vi "Write Value at Path(Array).vi"(8 "error in (no error)":errorcluster, 9 "Element in":variant, 10 "Path in":string[](array[string]), 11 "Variant in":variant) -> (0 "error out":errorcluster, 3 "Variant out":variant)   [LabVIEW 2020, in "Variant Data Manipulation.lvlib"]
uses:
  Variant Data Manipulation.lvlib
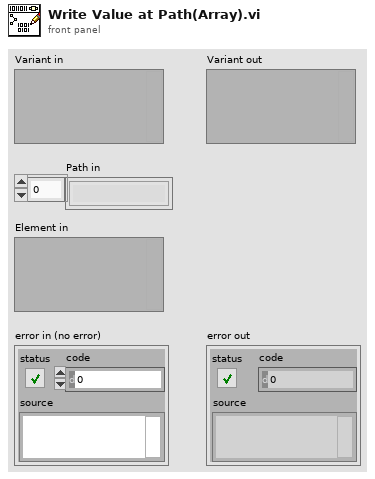
[diagram p1: front panel]
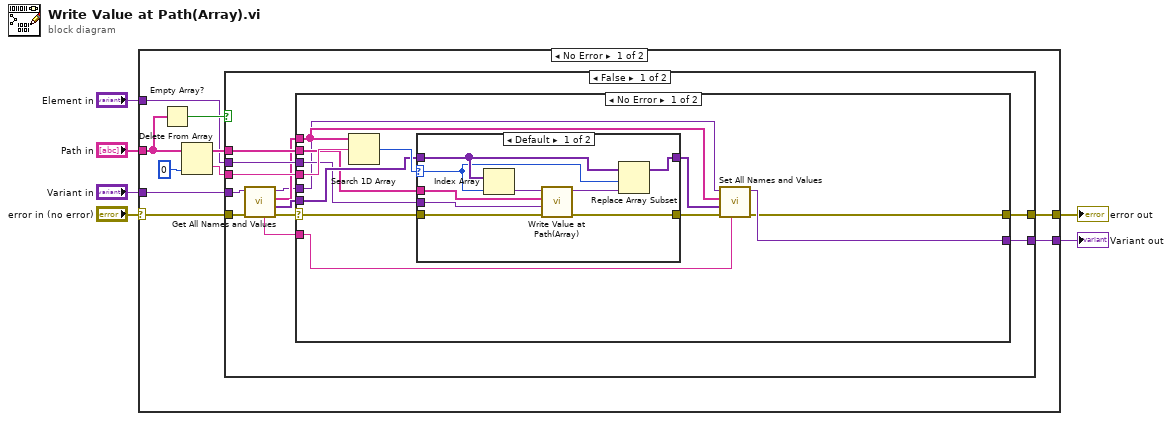
[diagram p0: block diagram]
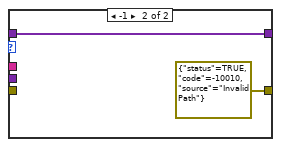
[diagram p2: hidden frame]
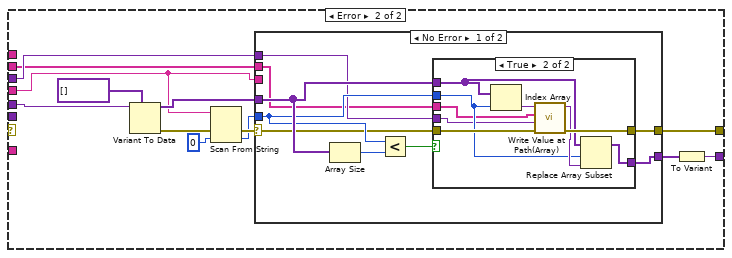
[diagram p3: hidden frame]
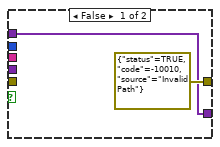
[diagram p4: hidden frame]
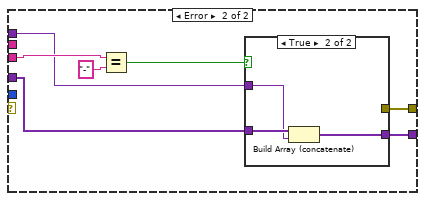
[diagram p5: hidden frame]
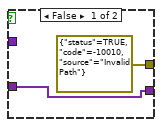
[diagram p6: hidden frame]
diagram:
  n1 = case shown="No Error" "error in (no error)" {
    selector: "error in (no error)" -> [w15 w101]
    tunnel: "Path in" -> [w11 _]
    tunnel: "Variant in" -> [w16 w100]
    tunnel: [w7 w101] -> w4
    tunnel: [w8 w100] -> w2
    tunnel: "Element in" -> [w9 _]
    frame No Error {
      n2 = Empty Array?(array=w11) -> (empty?=w10:bool)
      n3 = Delete From Array(array=w11, index=0) -> (deleted portion=w14:string, array with subset deleted=w12:string[])  [unwired: 1 in]
      n4 = case shown="False" w10 {
        tunnel: w16 -> [w28 _]
        tunnel: w15 -> [w27 w99]
        tunnel: w14 -> [w24 _]
        tunnel: w12 -> [w23 _]
        tunnel: w9 -> [w22 w98]
        tunnel: [w18 w98] -> w8
        tunnel: [w17 w99] -> w7
        frame False {
          n5 = call "Get All Names and Values.vi"("error in"=w27, "Cluster in"=w28) -> ("error out"=w26:errorcluster, "Values"=w25:variant[], "Element Names"=w21:string[], "Cluster out"=w20:variant, "Cluster Name"=w19:string)  [unwired: 5 in]
          n6 = case shown="No Error" w26 {
            selector: w26 -> [w39 _]
            tunnel: w20 -> [w29 w62]
            tunnel: w24 -> [w38 w53]
            tunnel: w21 -> [w34 _]
            tunnel: w25 -> [w40 _]
            tunnel: w23 -> [w37 w57]
            tunnel: w22 -> [w36 w58]
            tunnel: w19 -> [w35 _]
            tunnel: [w31 w56] -> w18
            tunnel: [w30 w54] -> w17
            frame No Error {
              n7 = Search 1D Array(1D array=w34, element=w38) -> (index of element=w41:i32)  [unwired: 1 in]
              n8 = case shown="Default" w41 {
                selector: w41 -> [w46 _]
                tunnel: [w48 errorcluster {"status"=TRUE, "code"=-10010, "source"="Invalid Path"} ("error IO")] -> w32
                tunnel: w40 -> [w47 w51]
                tunnel: w39 -> [w49 _]
                tunnel: w37 -> [w43 _]
                tunnel: w36 -> [w42 _]
                tunnel: [w44 w51] -> w33
                frame Default {
                  n9 = Index Array(array=w47, index=w46) -> (element=w50:variant)
                  n10 = call "Write Value at Path(Array).vi"("error in (no error)"=w49, "Element in"=w42, "Path in"=w43, "Variant in"=w50) -> ("error out"=w48:errorcluster, "Variant out"=w45:variant)  [unwired: 6 in]
                  n11 = Replace Array Subset(array=w47, new element=w45, index=w46) -> (w44:variant[])
                }
                frame -1 {
                }
              }
              n12 = call "Set All Names and Values.vi"("Cluster Name"=w35, "error in"=w32, "values"=w33, "Element Names"=w34, "Cluster in"=w29) -> ("error out"=w30:errorcluster, "Cluster out"=w31:variant)  [unwired: 5 in]
            }
            frame Error {
              n13 = Variant To Data(type=variant[] [], Variant=w62) -> (data=w60:variant[], error out=w59:errorcluster)  [unwired: 1 in]
              n14 = Scan From String(input string=w53, error in=w59, default 1=0 ("default value 1")) -> (error out=w64:errorcluster, output 1=w63:i32)  [unwired: 2 in, 2 out]
              n15 = case shown="No Error" w64 {
                selector: w64 -> [w68 _]
                tunnel: [w69 w92] -> w54
                tunnel: w63 -> [w72 _]
                tunnel: w60 -> [w73 w88]
                tunnel: [w74 w86] -> w55
                tunnel: w58 -> [w67 w87]
                tunnel: w57 -> [w66 _]
                tunnel: w53 -> [_ w91]
                frame No Error {
                  n16 = Array Size(array=w73) -> (size(s)=w71:i32)
                  n17 = Less?(x=w72, y=w71) -> (x < y?=w70:bool)
                  n18 = case shown="True" w70 {
                    tunnel: [w75 w82] -> w74
                    tunnel: w73 -> [w75 w80]
                    tunnel: w72 -> [_ w79]
                    tunnel: [errorcluster {"status"=TRUE, "code"=-10010, "source"="Invalid Path"} ("error IO") w83] -> w69
                    tunnel: w68 -> [_ w84]
                    tunnel: w67 -> [_ w77]
                    tunnel: w66 -> [_ w78]
                    frame False {
                    }
                    frame True {
                      n19 = Index Array(array=w80, index=w79) -> (element=w85:variant)
                      n20 = call "Write Value at Path(Array).vi"("error in (no error)"=w84, "Element in"=w77, "Path in"=w78, "Variant in"=w85) -> ("error out"=w83:errorcluster, "Variant out"=w81:variant)  [unwired: 6 in]
                      n21 = Replace Array Subset(array=w80, new element=w81, index=w79) -> (w82:variant[])
                    }
                  }
                }
                frame Error {
                  n22 = Equal?(x=w91, y="-") -> (x = y?=w89:bool)
                  n23 = case shown="True" w89 {
                    tunnel: [errorcluster {"status"=TRUE, "code"=-10010, "source"="Invalid Path"} ("error IO") _] -> w92
                    tunnel: w88 -> [w93 w97]
                    tunnel: w87 -> [_ w96]
                    tunnel: [w93 w95] -> w86
                    frame False {
                    }
                    frame True {
                      n24 = Build Array (concatenate)(w97, w96) -> (w95:variant[])
                    }
                  }
                }
              }
              n25 = To Variant(anything=w55) -> (Variant=w56:variant)
            }
          }
        }
        frame True {
        }
      }
    }
    frame Error {
    }
  }
  "error out" <- w4
  "Variant out" <- w2
